vi "ConfigureLevel.vi"(8 "error in (no error)":errorcluster, 11 "Keysight44xx in":refnum<class "Keysight44xx.lvclass">) -> (0 "error out":errorcluster, 3 "Keysight44xx out":refnum<class "Keysight44xx.lvclass">)   [LabVIEW 2018, in "SpecAnPlugins.lvlib" / "Keysight44xx.lvclass"]
doc: "This function configures the vertical attributes of the spectrum analyzer. This corresponds to the Amplitude Units, Input Attenuation, Input Impedance, Reference Level, and Reference Level Offset attributes."
uses:
  Keysight44xx.lvclass
  C:/Users/ico/Documents/Projects/NistPluggableModules/SpecAn/SpecAnPlugins/SpecAnBaseClass/SpecAnBase.lvclass
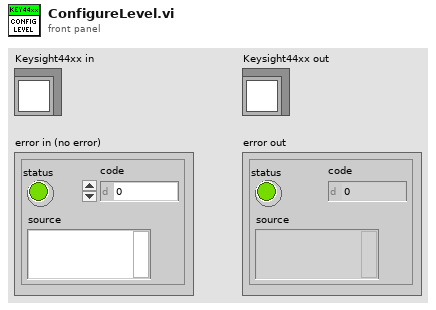
[diagram p1: front panel]
types:
  T1 = typedef "SpecAnPlugins.lvlib/SpecAnBase.lvclass/Acquisition.ctl" = cluster{"Handle":string, "Connected":bool, "Enabled":bool, "SweepModeContinuous":bool, "NumberOfSweeps":i32, "DetectorTypeAuto":bool, "DetectorType":i32, "VerticalScale":i32, "MaximumTime(seconds)":dbl}
  T2 = typedef "SpecAnPlugins.lvlib/SpecAnBase.lvclass/Level.ctl" = cluster{"InputImpedance":dbl, "AttenuationAuto":bool, "ReferenceLevel":dbl, "Attenuation":dbl, "ReferenceLevelOffset":dbl, "amplitude units (dBm)":i32}
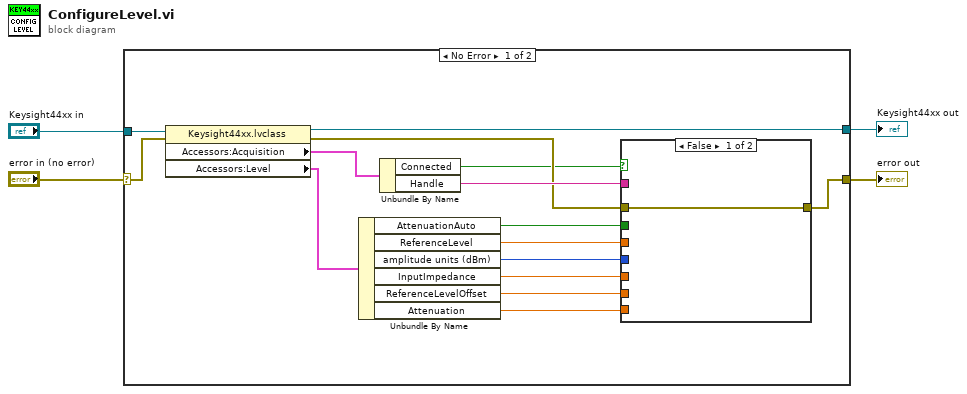
[diagram p0: block diagram]
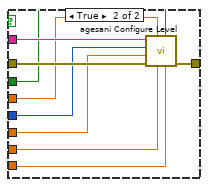
[diagram p2: hidden frame]
diagram:
  n1 = case shown="No Error" "error in (no error)" {
    selector: "error in (no error)" -> [w18 w31]
    tunnel: [w8 w31] -> w3
    tunnel: "Keysight44xx in" -> [w19 w30]
    tunnel: [w15 w30] -> w1
    frame No Error {
      n2 = property class="Keysight44xx.lvclass"(reference=w19, error in=w18) -> (reference out=w15:refnum<class "Keysight44xx.lvclass">, error out=w14:errorcluster, "Accessors:Acquisition"=w17:T1, "Accessors:Level"=w7:T2)
      n3 = Unbundle By Name(w7) -> ("AttenuationAuto"=w13:bool, "ReferenceLevel"=w12:dbl, "amplitude units (dBm)"=w6:i32, "InputImpedance"=w11:dbl, "ReferenceLevelOffset"=w10:dbl, "Attenuation"=w9:dbl)
      n4 = Unbundle By Name(w17) -> ("Connected"=w5:bool, "Handle"=w16:string)
      n5 = case shown="False" w5 {
        tunnel: w16 -> [_ w29]
        tunnel: w14 -> [w20 w28]
        tunnel: w13 -> [_ w27]
        tunnel: w12 -> [_ w26]
        tunnel: w11 -> [_ w25]
        tunnel: w10 -> [_ w24]
        tunnel: w9 -> [_ w23]
        tunnel: [w20 w22] -> w8
        tunnel: w6 -> [_ w21]
        frame False {
        }
        frame True {
          n6 = call <instrlib>:"agesani Configure Level.vi"("attenuation (10.0)"=w23, "attenuation auto (On)"=w27, "reference level offset (0.0)"=w24, "reference level (0.0)"=w26, "error in (no error)"=w28, "input impedance (50.0)"=w25, "amplitude units (dBm)"=w21, "instrument handle"=w29) -> ("error out"=w22:errorcluster)  [unwired: 3 out]
        }
      }
    }
    frame Error {
    }
  }
  "error out" <- w3
  "Keysight44xx out" <- w1
